vi "Monitor Spectrum Display Setup.vi"(0 "VISA resource name":refnum<visa-resource-name>, 7 "Y-Axis Scale Per Division (10 dB)":dbl=10.0 format="%^#_6g", 9 "Y-Axis Reference Level (-45 dB)":dbl=-45.0 format="%^#_6g", 11 "error in (no error)":errorcluster) -> (4 "VISA resource name out":refnum<visa-resource-name>, 15 "error out":errorcluster)   [LabVIEW 2014, in "Agilent ESA PSA Series.lvlib"]
doc: "Configures the Monitor Spectrum display of the Noise Figure personality.\n\n<B>Note:</B> \n\nThis VI is only valid in Noise Figure personality. Use <B>Switch Personality</B> VI to switch to Noise Figure before calling this VI."
uses:
  Agilent ESA PSA Series.lvlib
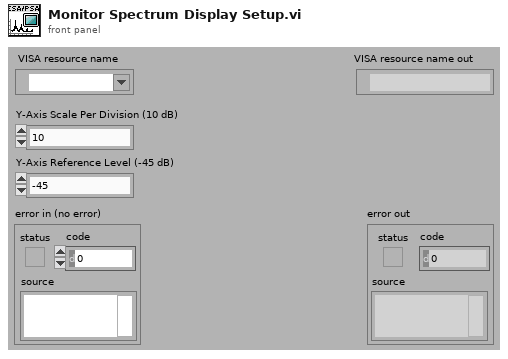
[diagram p1: front panel]
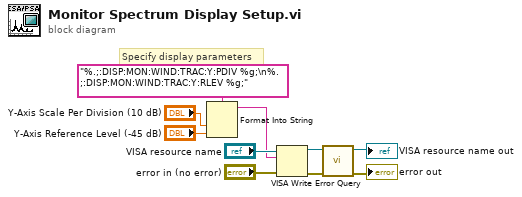
[diagram p0: block diagram]
diagram:
  # "Specify display parameters"
  n1 = Format Into String(format string="%.;:DISP:MON:WIND:TRAC:Y:PDIV %g;\n%.;:DISP:MON:WIND:TRAC:Y:RLEV %g;", "Y-Axis Scale Per Division (10 dB)", "Y-Axis Reference Level (-45 dB)") -> (resulting string=w1:string)  [unwired: 2 in, 1 out]
  n2 = VISA Write(VISA resource name="VISA resource name", write buffer=w1, error in (no error)="error in (no error)") -> (VISA resource name out=w8:refnum<visa-resource-name>, error out=w7:errorcluster)  [unwired: 1 out]
  n3 = call "Error Query.vi"("error in (no error)"=w7, "VISA resource name"=w8) -> ("error out"=→"error out":errorcluster, "VISA resource name out"=→"VISA resource name out":refnum<visa-resource-name>)  [unwired: 6 in, 2 out]
